vi "Create Counter.vi"(8 "error in (no error)":errorcluster) -> (0 "error out":errorcluster, 2 "Counter Updated event for registration":refnum<user-event>, 3 "Counter out":refnum<class "Counter.lvclass">)   [LabVIEW 2018, in "Counter.lvclass"]
uses:
  Counter.lvclass
  Counter.lvclass/Counter.ctl
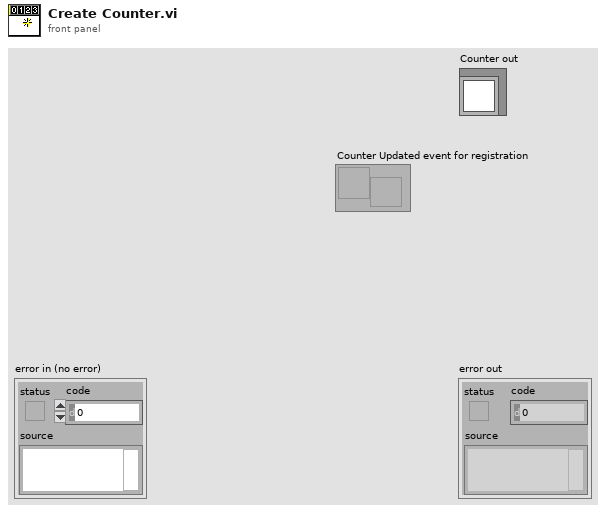
[diagram p1: front panel]
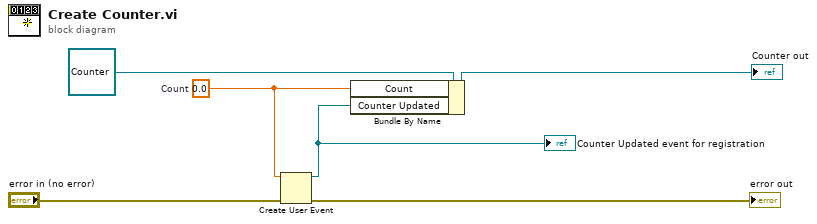
[diagram p0: block diagram]
diagram:
  w4 = 0.0  # Count
  n1 = Create User Event(user event datatype=w4, error in="error in (no error)") -> (user event=w3:refnum<user-event>, error out=→"error out":errorcluster)
  "Counter Updated event for registration" <- w3
  n2 = Bundle By Name(cluster=refnum<class "Counter.lvclass"> refnum ("Counter in"), "Count"=w4, "Counter Updated"=w3) -> (→"Counter out":refnum<class "Counter.lvclass">)
